vi "OxfordTests2.vi"() -> ()   [LabVIEW 2021]
uses:
  <instrlib>/Mercury iXX/Public/Controls/Comms Transport Layer.ctl
  <instrlib>/Mercury iXX/Public/Controls/Serial Settings.ctl
  <instrlib>/Mercury iXX/Public/Controls/ISOBus Address.ctl
  <instrlib>/Mercury iXX/Public/Libraries/System/Open/Open System.vi
  <instrlib>/Mercury iXX/Public/Libraries/System/Read/Catalogue (Read).vi
  <instrlib>/Mercury iXX/Mercury iXX.lvlib
  <instrlib>/Mercury iXX/Public/Libraries/System.lvlib
panel:
  out "Device Details":T1
  in  "Connection Details":T5={"VISA resource name"="", "Comms Layer"=enum."Ethernet TCP/IP", "IP Address"="", "Serial Configuration"={"Baud Rate"=9600, "Parity"=0, "Data Bits"=8, "Stop Bits"=10, "Flow Control"=0}, "ISOBUS address"=-1} {"Serial Configuration"."Flow Control" items=["None", "XON/XOFF", "RTS/CTS", "XON/XOFF & RTS/CTS", "DTR/DSR", "XON/XOFF & DTR/DSR"]; "Serial Configuration"."Stop Bits" items=["1.0"=10, "2.0"=20]; "Serial Configuration"."Data Bits" items=["7"=7, "8"=8]; "Serial Configuration"."Parity" items=["None", "Odd", "Even"]; "Serial Configuration"."Baud Rate" items=["300"=300, "600"=600, "1200"=1200, "2400"=2400, "4800"=4800, "9600"=9600, "19200"=19200]}
  in  "Clear Previous Connections (False)":bool
  in  "ID Query (True)":bool=TRUE
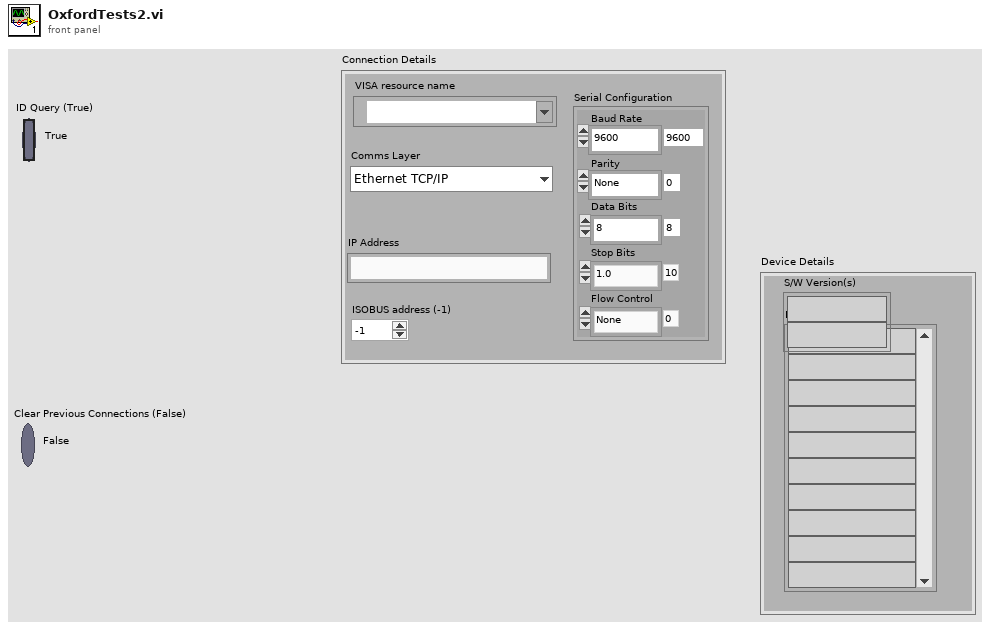
[diagram p1: front panel]
types:
  T1 = cluster{"Devices":string[], "S/W Version(s)":string[]}
  T2 = typedef "Mercury iXX.lvlib/Comms Transport Layer.ctl" = enum16{"Ethernet TCP/IP", "USB", "ISOBus - RS-232", "GPIB"}
  T3 = typedef "Mercury iXX.lvlib/Serial Settings.ctl" = cluster{"Baud Rate":u32, "Parity":u16, "Data Bits":u16, "Stop Bits":u16, "Flow Control":u16}
  T4 = typedef "Mercury iXX.lvlib/ISOBus Address.ctl" = i32
  T5 = cluster{"VISA resource name":refnum<visa-resource-name>, "Comms Layer":T2, "IP Address":string, "Serial Configuration":T3, "ISOBUS address":T4}
  T6 = typedef "Mercury iXX.lvlib/Mercury Reference.ctl" = cluster{"Comms":refnum<visa-resource-name>, "Device ID":string[], "Comms Layer":T2, "Command":string, "Query reference":T7}
  T7 = typedef "Mercury iXX.lvlib/Query Dynamic Reference.ctl" = refnum<vi>
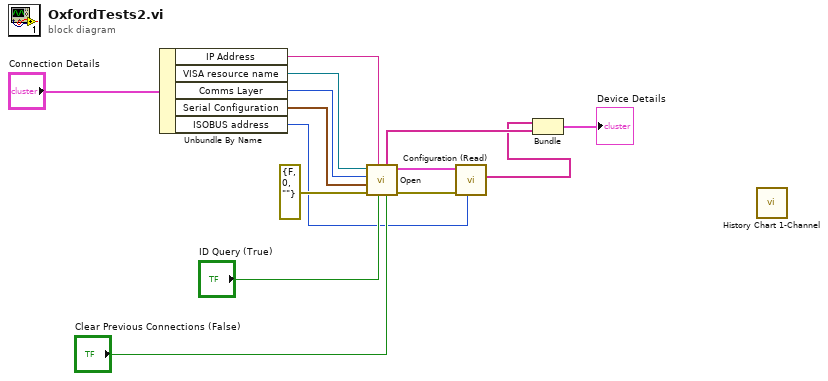
[diagram p0: block diagram]
diagram:
  n1 = Unbundle By Name("Connection Details") -> ("IP Address"=w6:string, "VISA resource name"=w5:refnum<visa-resource-name>, "Comms Layer"=w4:T2, "Serial Configuration"=w8:T3, "ISOBUS address"=w7:T4)
  n2 = call-poly <instrlib>:"Open.vi"("Clear Previous Connections (False)"="Clear Previous Connections (False)", "ID Query (True)"="ID Query (True)", "IP Address"=w6, "error in (no error)"=errorcluster {"status"=FALSE, "code"=0, "source"=""}, "Serial Configuration"=w8, "Comms Layer"=w4, "VISA resource name"=w5) -> ("error out"=w10:errorcluster, "Mercury Reference Out"=w11:T6, "S/W Version(s)"=w3:string[])  [unwired: 2 out]
  n3 = call-poly <instrlib>:"Configuration (Read).vi"("ISOBUS address"=w7, "error in"=w10, "Mercury Reference In"=w11) -> ("Devices"=w1:string[])  [unwired: 8 out]
  n4 = Bundle("Devices"=w1, "S/W Version(s)"=w3) -> (→"Device Details":T1)  [unwired: 1 out]
  n5 = call <userlib>:"History Chart 1-Channel.vi"() -> ()  [unwired: 1 in]
